vi "Torque_.vi"(5 "gap":dbl, 6 "input_speed":dbl) -> (1 "Torque":dbl, 2 "appended array":dbl[](array[numeric]))   [LabVIEW 2013]
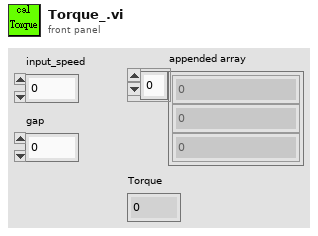
[diagram p1: front panel]
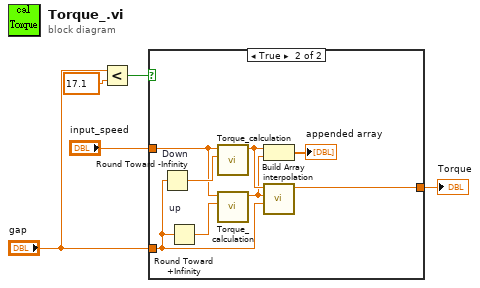
[diagram p0: block diagram]
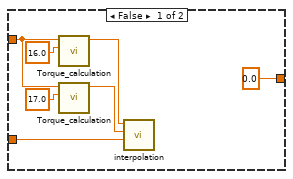
[diagram p2: hidden frame]
diagram:
  n1 = Less?(x="gap", y=17.1) -> (x < y?=w4:bool)
  n2 = case shown="True" w4 {
    tunnel: "gap" -> [w7 w20]
    tunnel: "input_speed" -> [w11 w18]
    tunnel: [0.0 ("Output") w16] -> w2
    frame False {
      n3 = call "Torque_calculation.vi"("Position"=16.0, "speed"=w11) -> ("Torque"=w9:dbl)  [unwired: 9 in]
      n4 = call "Torque_calculation.vi"("Position"=17.0, "speed"=w11) -> ("Torque"=w8:dbl)  [unwired: 9 in]
      n5 = call "interpolation.vi"("position"=w7, "Up"=w8, "Down"=w9) -> ()  [unwired: 8 in, 1 out]
    }
    frame True {
      n6 = Round Toward -Infinity "Down"(1:w20) -> (0:w19:dbl)
      n7 = Round Toward +Infinity "up"(x=w20) -> (ceil(x): smallest int >= x=w17:dbl)
      n8 = call "Torque_calculation.vi"("Position"=w19, "speed"=w18) -> ("Torque"=w15:dbl)  [unwired: 9 in]
      n9 = call "Torque_calculation.vi"("Position"=w17, "speed"=w18) -> ("Torque"=w14:dbl)  [unwired: 9 in]
      n10 = Build Array(w15, w14) -> (→"appended array":dbl[])
      n11 = call "interpolation.vi"("position"=w20, "Up"=w14, "Down"=w15) -> ("Output"=w16:dbl)  [unwired: 8 in]
    }
  }
  "Torque" <- w2
